vi "Init Module.vi"(8 "error in (no error)":errorcluster, 11 "Singleton Module Admin in":refnum<class "Delacor_lib_QMH_Module Admin.lvclass">) -> (0 "error out":errorcluster, 2 "Tool Module Request Events":T1, 3 "Singleton Module Admin out":refnum<class "Delacor_lib_QMH_Module Admin.lvclass">)   [LabVIEW 2015, in "Tool Module.lvlib"]
doc: "Initialize the module by creating Broadcast Events, Request Events, and synchronization rendezvous.\n_____\nBased on Delacor QMH Project Template 2.1.0.2."
uses:
  Tool Module.lvlib
  <vilib>/Delacor/Delacor QMH/Libraries/Module Admin_class/Delacor_lib_QMH_Module Admin.lvclass
  Request Events--cluster.ctl
  Stop Argument--cluster.ctl
  Get Module Execution Status Argument--cluster.ctl
  Show Diagram Argument--cluster.ctl
  Test Trig 2 Argument--cluster.ctl
  Support/Timer Setup Params Typedef.ctl
  GOTO Argument--cluster.ctl
  Support/_GoTo Cmd Typedef--enum.ctl
  Start Inspect Argument--cluster.ctl
  Support/_Sample Data Rtn Cluster--typedef.ctl
  CONNECT Argument--cluster.ctl
  Get All Inspect Data Argument--cluster.ctl
  Get All Inspect Data (Reply Payload)--cluster.ctl
  Get Inspection Limits Argument--cluster.ctl
  Get Inspection Limits (Reply Payload)--cluster.ctl
  Set Inspection Limits Argument--cluster.ctl
  Support/_Inspection Limits cluster--typedef.ctl
  Update Status Argument--cluster.ctl
  Start Data Monitor Argument--cluster.ctl
  Get FPGA Setup Params Argument--cluster.ctl
  Get FPGA Setup Params (Reply Payload)--cluster.ctl
  Tool Typedefs/_FPGA Setup Params Cluster--typedef.ctl
  Tool Typedefs/_FPGA Timing Constraints Cluster--typedef.ctl
  Tool Typedefs/_FPGA Timing Ctrl Cluster--typedef.ctl
  Tool Typedefs/_FPGA Laser Config Cluster--typedef.ctl
  Tool Typedefs/_FPGA Peak Proc Cfg Cluster--typedef.ctl
  Tool Typedefs/_FPGA SPI Cfg Cluster--typedef.ctl
  Set FPGA Setup Params Argument--cluster.ctl
  Set Tool Config Argument--cluster.ctl
  Tool Config/_Configuration Cluster_v3--typedef.ctl
  Tool Config/_Tool Block Cluster_v3--typedef.ctl
  Tool Config/_Motor Block Cluster_v2--typedef.ctl
  Tool Config/_Verification Blk Cluster--typedef.ctl
  Tool Config/_ProbeConfigParams Cluster--typedef.ctl
  Tool Config/_Sensor Block Cluster--typedef.ctl
  Tool Config/_SensorConfigParams Cluster--typedef.ctl
  Get Tool Config Argument--cluster.ctl
  Get Tool Config (Reply Payload)--cluster.ctl
  Set Integration Count Argument--cluster.ctl
  Set Laser Params Argument--cluster.ctl
  Get Mtrl Ctrl Reg Argument--cluster.ctl
  Get Mtrl Ctrl Reg (Reply Payload)--cluster.ctl
  Commit Ctrl Reg Argument--cluster.ctl
  Set Event Logger Argument--cluster.ctl
  Event Logger Library/Event Log/EventLog.lvclass
  Write to File Argument--cluster.ctl
  Read from File Argument--cluster.ctl
  Set Device Temp Thresholds Argument--cluster.ctl
  Tool Typedefs/_Temperature Threshold Arrays--typedef.ctl
  Get Cycle Count Argument--cluster.ctl
  Get Cycle Count (Reply Payload)--cluster.ctl
  Tool Config/Tool Cfg.lvlib
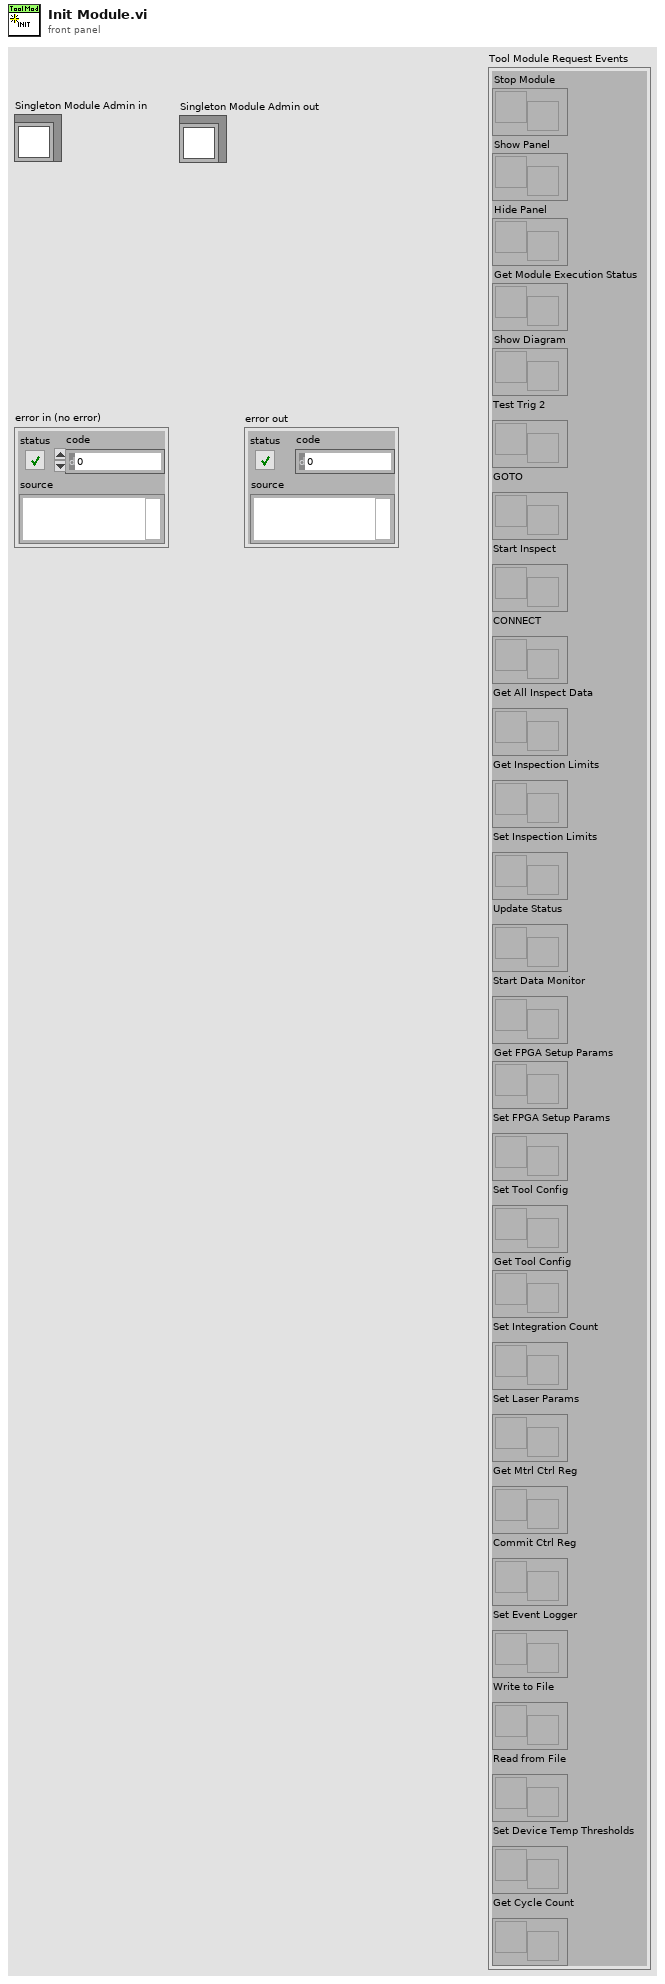
[diagram p1: front panel]
types:
  T1 = typedef "Tool Module.lvlib/Request Events--cluster.ctl" = cluster{"Stop Module":refnum<user-event>, "Show Panel":refnum<user-event>, "Hide Panel":refnum<user-event>, "Get Module Execution Status":refnum<user-event>, "Show Diagram":refnum<user-event>, "Test Trig 2":refnum<user-event>, "GOTO":refnum<user-event>, "Start Inspect":refnum<user-event>, "CONNECT":refnum<user-event>, "Get All Inspect Data":refnum<user-event>, "Get Inspection Limits":refnum<user-event>, "Set Inspection Limits":refnum<user-event>, "Update Status":refnum<user-event>, "Start Data Monitor":refnum<user-event>, "Get FPGA Setup Params":refnum<user-event>, "Set FPGA Setup Params":refnum<user-event>, "Set Tool Config":refnum<user-event>, "Get Tool Config":refnum<user-event>, "Set Integration Count":refnum<user-event>, "Set Laser Params":refnum<user-event>, "Get Mtrl Ctrl Reg":refnum<user-event>, "Commit Ctrl Reg":refnum<user-event>, "Set Event Logger":refnum<user-event>, "Write to File":refnum<user-event>, "Read from File":refnum<user-event>, "Set Device Temp Thresholds":refnum<user-event>, "Get Cycle Count":refnum<user-event>}
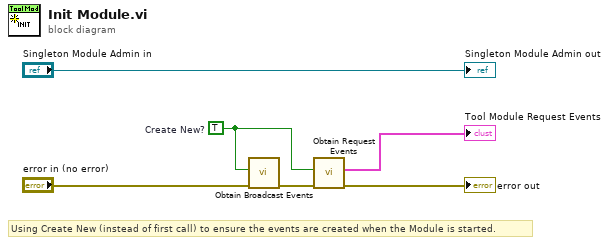
[diagram p0: block diagram]
diagram:
  w3 = TRUE  # Create New?
  # "Using Create New (instead of first call) to ensure the events are created when the Module is started."
  n1 = call "Obtain Broadcast Events.vi"("error in (no error)"="error in (no error)", "Create New?"=w3) -> ("error out"=w6:errorcluster)  [unwired: 8 in, 1 out]
  n2 = call "Obtain Request Events.vi"("error in (no error)"=w6, "Create New?"=w3) -> ("error out"=→"error out":errorcluster, "Tool Module Request Events"=→"Tool Module Request Events":T1)  [unwired: 8 in]
  "Singleton Module Admin out" <- "Singleton Module Admin in"
